vi "Sea-Level SWI Initialize.vi"(8 "error in (no error)":errorcluster, 11 "Configuration":T2={"BusType"=enum."PCI/ISA/PCMCIA", "Card"=0, "USB"=16, "IP"=0, "COM"=1, "Baud Rate"=enum."9600"}) -> (0 "error out":errorcluster {"code" format="%.0x"}, 3 "Handle Out":i32, 5 "Sea-Level SWI":T1)   [LabVIEW 2011]
uses:
  TypeDefs/Sea-Level SWI Configuration.ctl
  TypeDefs/Sea-Level SWI Adapter Info.ctl
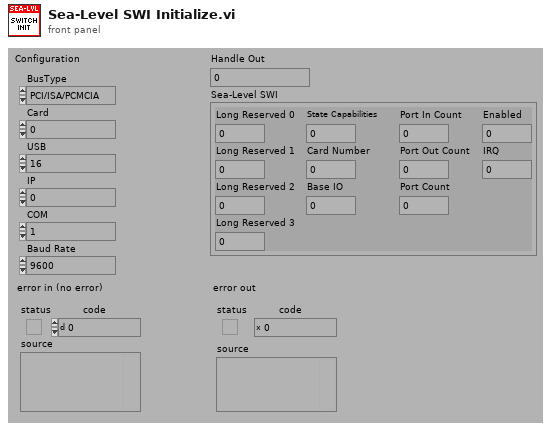
[diagram p1: front panel]
types:
  T1 = typedef "Sea-Level SWI Adapter Info.ctl" = cluster{"Long Reserved 0":i32, "Long Reserved 1":i32, "Long Reserved 2":i32, "Long Reserved 3":i32, "State Capabilities":i32, "Card Number":i16, "Base IO":i16, "Port In Count":i8, "Port Out Count":i8, "Port Count":i8, "Enabled":i8, "IRQ":i16}
  T2 = typedef "Sea-Level SWI Configuration.ctl" = cluster{"BusType":enum32{"PCI/ISA/PCMCIA", "USB", "Ethernet", "Serial"}, "Card":i32, "USB":i32, "IP":u32, "COM":i32, "Baud Rate":enum16{"300", "600", "1200", "2400", "4800", "9600"}}
  T3 = enum32{"PCI/ISA/PCMCIA", "USB", "Ethernet", "Serial"}
  T4 = enum16{"300", "600", "1200", "2400", "4800", "9600"}
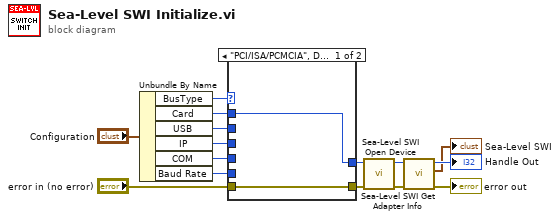
[diagram p0: block diagram]
diagram:
  n1 = Unbundle By Name("Configuration") -> ("BusType"=w14:T3, "Card"=w13:i32, "USB"=w12:i32, "IP"=w11:u32, "COM"=w10:i32, "Baud Rate"=w1:T4)
  n2 = case shown="\"PCI/ISA/PCMCIA\", Default" w14 {
    tunnel: "error in (no error)" -> [w17 w18]
    tunnel: w13 -> [w16 _]
    tunnel: w12 -> [_ _]
    tunnel: w11 -> [_ _]
    tunnel: w10 -> [_ _]
    tunnel: [w17 w18] -> w3
    tunnel: [w16 _] -> w4
    tunnel: w1 -> [_ _]
    frame "PCI/ISA/PCMCIA", Default {
    }
    frame "USB".."Serial" {
    }
  }
  n3 = call "Sea-Level SWI Open Device.vi"("error in (no error)"=w3, "Card Number"=w4) -> ("error out"=w7:errorcluster, "Handle Out"=w6:i32)  [unwired: 8 out]
  n4 = call "Sea-Level SWI Get Adapter Info.vi"("error in (no error)"=w7, "Handle"=w6) -> ("error out"=→"error out":errorcluster, "Adapter Info"=→"Sea-Level SWI":T1, "Handle Out"=→"Handle Out":i32)  [unwired: 7 out]
